vi "Lead Screw Control.vi"() -> ()   [LabVIEW 2012]
uses:
  Robot Global Data.vi
panel:
  out "front":bool
  out "rear":bool
  out "x-y":dbl
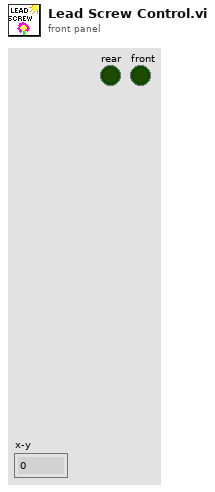
[diagram p1: front panel]
types:
  T1 = typedef "WPI_MotorControlDeviceRef.ctl" = cluster{"DeviceStatus":errorcluster, "Type":enum16{"PWM", "CAN"}, "PWM":cluster{"Digital Module":T2, "PWM Channel":T3, "DeadBand":T4}, "CAN":cluster{"Device Number":u8, "Control Mode":T5, "Semaphore":T6, "Max Vout":dbl}, "Invert":bool, "TransformRef":T7, "InvTransformRef":T7}
  T2 = typedef "FPGA_TypedefDigitalModule.ctl" = enum16{"Digital Module 1", "Digital Module 2"}
  T3 = typedef "FPGA_DIOPWMChannel.ctl" = enum8{"PWM 1", "PWM 2", "PWM 3", "PWM 4", "PWM 5", "PWM 6", "PWM 7", "PWM 8", "PWM 9", "PWM 10", "Invalid"}
  T4 = typedef "WPI_PWMDeadband.ctl" = cluster{"Name":string, "maxPositivePwm":i32, "minPositivePwm":i32, "centerPwm":i32, "maxNegativePwm":i32, "minNegativePwm":i32, "angularRange":u16}
  T5 = typedef "WPI_CANJaguar_ControlMode.ctl" = enum8{"Percent VBus", "Current", "Speed", "Position", "Voltage"}
  T6 = typedef "Semaphore RefNum" = refnum<k1>
  T7 = typedef "WPI_PWMTransform_ConPane.ctl" = refnum<vi>
  T8 = typedef "WPI_DigitalInputDevRef.ctl" = cluster{"DevStatus":errorcluster, "DIO Channel":T9, "Digital Module":T2}
  T9 = typedef "FPGA_DIOChannel.ctl" = enum8{"DIO 1", "DIO 2", "DIO 3", "DIO 4", "DIO 5", "DIO 6", "DIO 7", "DIO 8", "DIO 9", "DIO 10", "DIO 11", "DIO 12", "DIO 13", "DIO 14", "Invalid"}
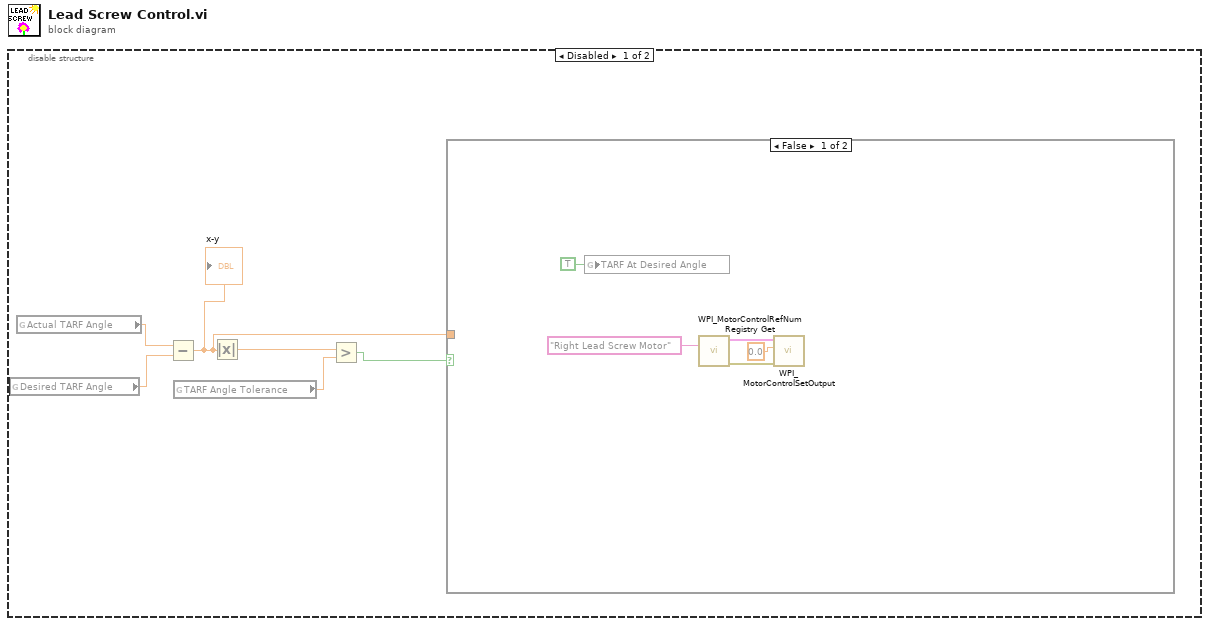
[diagram p0: block diagram]
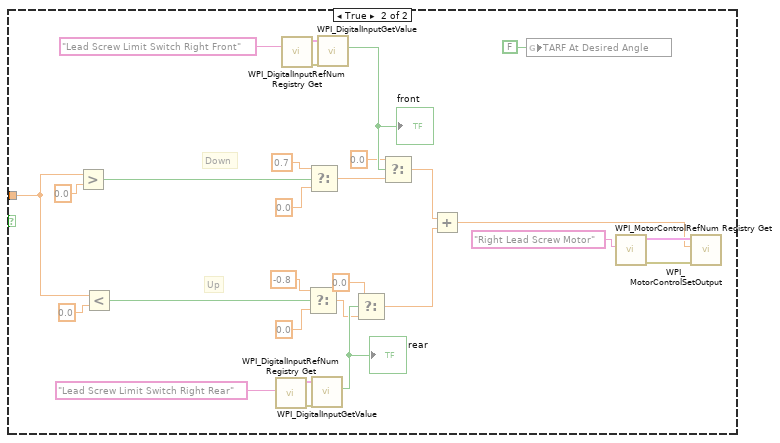
[diagram p2: hidden frame]
diagram:
  n1 = disable-structure shown="Disabled" {
    frame Disabled {
      n2 = global read "Robot Global Data.vi" "Desired TARF Angle"() -> (w3:dbl)
      n3 = global read "Robot Global Data.vi" "Actual TARF Angle"() -> (w4:dbl)
      n4 = Subtract(x=w4, y=w3) -> (x-y=w1:dbl)
      "x-y" <- w1
      n5 = global read "Robot Global Data.vi" "TARF Angle Tolerance"() -> (w5:dbl)
      n6 = Absolute Value(x=w1) -> (abs(x)=w6:dbl)
      n7 = Greater?(x=w6, y=w5) -> (0:w2:bool)
      n8 = case shown="False" w2 {
        tunnel: w1 -> [_ w39]
        frame False {
          n9 = global write "Robot Global Data.vi" "TARF At Desired Angle"(TRUE ("TARF At Desired Angle")) -> ()
          n10 = call <vilib>:"WPI_MotorControlRefNum Registry Get.vi"("refnum name"="Right Lead Screw Motor") -> ("error out"=w8:errorcluster, "MotorControlDevRef"=w9:T1)  [unwired: 9 in]
          n11 = call <vilib>:"WPI_MotorControlSetOutput.vi"("error in (no error)"=w8, "Output"=0.0, "MotorControlDevRef"=w9) -> ()  [unwired: 6 in, 3 out]
        }
        frame True {
          # "Up"
          # "Down"
          n12 = Greater?(x=w39, y=0.0) -> (0:w15:bool)
          n13 = Less?(x=w39, y=0.0) -> (x < y?=w14:bool)
          n14 = call <vilib>:"WPI_DigitalInputRefNum Registry Get.vi"("refnum name"="Lead Screw Limit Switch Right Rear") -> ("error out"=w24:errorcluster, "DigitalInputDevRef"=w23:T8)  [unwired: 9 in]
          n15 = call <vilib>:"WPI_DigitalInputRefNum Registry Get.vi"("refnum name"="Lead Screw Limit Switch Right Front") -> ("error out"=w28:errorcluster, "DigitalInputDevRef"=w27:T8)  [unwired: 9 in]
          n16 = Select(t=-0.8, s=w14, f=0.0) -> (s? t:f=w18:dbl)
          n17 = Select(t=0.7, s=w15, f=0.0) -> (s? t:f=w20:dbl)
          n18 = call <vilib>:"WPI_DigitalInputGetValue.vi"("error in (no error)"=w24, "DigitalInputDevRef"=w23) -> ("Value"=w21:bool)  [unwired: 7 in, 2 out]
          "rear" <- w21
          n19 = call <vilib>:"WPI_DigitalInputGetValue.vi"("error in (no error)"=w28, "DigitalInputDevRef"=w27) -> ("Value"=w26:bool)  [unwired: 7 in, 2 out]
          "front" <- w26
          n20 = Select(t=0.0 ("f"), s=w21, f=w18) -> (s? t:f=w30:dbl)
          n21 = Select(t=0.0, s=w26, f=w20) -> (s? t:f=w29:dbl)
          n22 = Add(x=w29, y=w30) -> (x+y=w35:dbl)
          n23 = global write "Robot Global Data.vi" "TARF At Desired Angle"(FALSE ("TARF At Desired Angle")) -> ()
          n24 = call <vilib>:"WPI_MotorControlRefNum Registry Get.vi"("refnum name"="Right Lead Screw Motor") -> ("error out"=w36:errorcluster, "MotorControlDevRef"=w37:T1)  [unwired: 9 in]
          n25 = call <vilib>:"WPI_MotorControlSetOutput.vi"("error in (no error)"=w36, "Output"=w35, "MotorControlDevRef"=w37) -> ()  [unwired: 6 in, 3 out]
        }
      }
    }
    frame Enabled {
    }
  }
